vi "ConvertMatBrgToPicture.vi"(8 "ErrorIn":errorcluster, 11 "CvMatIn":refnum<k24>) -> (0 "ErrorOut":errorcluster, 2 "NewPicture":picture, 3 "CvMatOut":refnum<k24>)   [LabVIEW 2021]
uses:
  C:/Localdata/Projects/TriekselSoft/TriekselsoftApplicationFramework/Source/.Externals/Library_EmguCV/Emgu.CV.Platform.NetStandard.dll
  Emgu.CV.Platform.NetStandard.dll
  <vilib>/picture/picture.llb/Draw True-Color Pixmap.vi
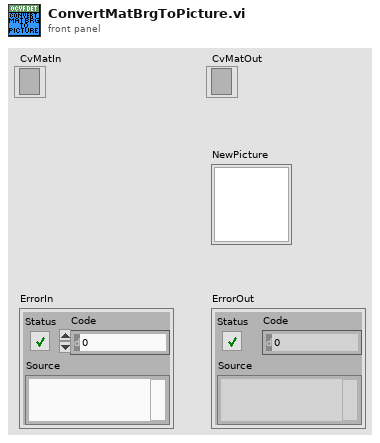
[diagram p1: front panel]
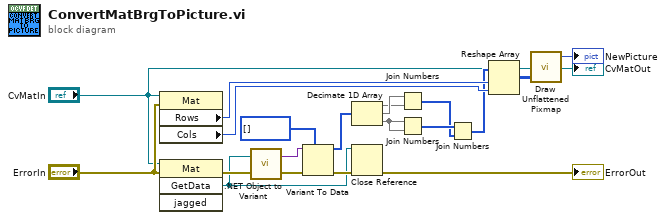
[diagram p0: block diagram]
diagram:
  n1 = property class="Mat"(reference="CvMatIn", error in="ErrorIn") -> ("Rows"=w13:i32, "Cols"=w12:i32)  [unwired: 2 out]
  n2 = invoke class="Mat" method="GetData"(reference="CvMatIn", error in="ErrorIn") -> (error out=w20:errorcluster, "GetData"=w10:refnum<k24>)  [unwired: 2 in, 2 out]
  n3 = call <vilib>:".NET Object to Variant.vi"("error in (no error)"=w20, ".NET object"=w10) -> ("error out"=w19:errorcluster, "variant"=w14:variant)
  n4 = Variant To Data(error in=w19, type=u8[] [], Variant=w14) -> (data=w11:u8[], error out=w18:errorcluster)
  n5 = Decimate 1D Array(w11) -> (w5:u8[], w6:u8[], w7:u8[])
  n6 = Close Reference(reference=w10, error in (no error)=w18) -> (error out=→"ErrorOut":errorcluster)
  n7 = Join Numbers(hi=w6, lo=w5) -> ((hi.lo)=w3:u16[])
  n8 = Join Numbers(hi=w7, lo=w7) -> ((hi.lo)=w4:u16[])
  n9 = Join Numbers(hi=w4, lo=w3) -> ((hi.lo)=w9:u32[])
  n10 = Reshape Array(w9, w13, w12) -> (w8:u32[][])
  n11 = call-poly <vilib>:"Draw Unflattened Pixmap.vi"("data (RGB format)"=w8) -> ("new picture"=→"NewPicture":picture)  [unwired: 8 in]
  "CvMatOut" <- "CvMatIn"
